vi "sv_Get Positive and Negative Max.vi"(11 "data":dbl[](array[numeric]) format="%.2f") -> (0 "negative index":i32, 1 "negative max":dbl format="%.2f", 2 "positive index":i32, 3 "positive max":dbl format="%.2f", 4 "absolute max":dbl format="%.2f", 6 "abs max index":i32)   [LabVIEW 2017, in "SoundVib_Transient.lvlib"]
uses:
  <vilib>/addons/Sound and Vibration/svt_Transients/SoundVib_Transient.lvlib
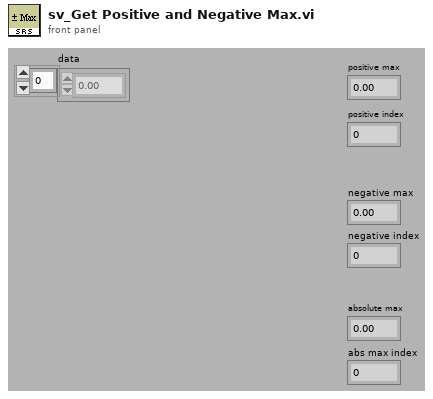
[diagram p1: front panel]
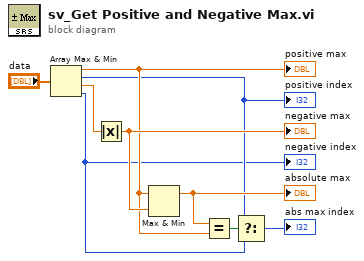
[diagram p0: block diagram]
diagram:
  n1 = Array Max & Min(array="data") -> (max value=w5:dbl, max index (indices)=w3:i32, min value=w8:dbl, min index (indices)=w2:i32)
  "positive max" <- w5
  "positive index" <- w3
  "negative index" <- w2
  n2 = Absolute Value(x=w8) -> (abs(x)=w7:dbl)
  "negative max" <- w7
  n3 = Max & Min(x=w5, y=w7) -> (max(x,y)=w6:dbl)  [unwired: 1 out]
  "absolute max" <- w6
  n4 = Equal?(x=w6, y=w5) -> (x = y?=w4:bool)
  n5 = Select(t=w3, s=w4, f=w2) -> (s? t:f=→"abs max index":i32)
